vi "CleanHandler.ProcDestructor.vi"(0 "i ref in":refnum<vi>, 3 "ms timeout (100)":i32=100, 5 "error in (no error)":errorcluster) -> (14 "i ref out":refnum<vi>, 17 "timed out":bool, 19 "error out":errorcluster)   [LabVIEW 2014, in "CleanHandler.lvlib"]
doc: "This is the counterpart to ProcConstructor and is called befor the \"deactivate\" is called. This can be used to shutdown/deinitialize things."
uses:
  CleanHandler.lvlib
  CSCore/CSSystem/CoreDefs/CoreDefs.error_type.ctl
  CSCore/CSSystem/CoreLib/CoreLib.string 2 byte array.vi
  CSCore/CSSystem/CoreLib/CoreLib.lvlib
  CSCore/BaseProcess/BaseProcess.lvlib
  CSCore/CSSystem/CSSystemLib/CSSystemLib.lvlib
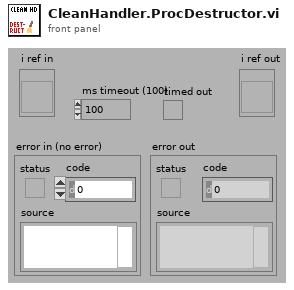
[diagram p1: front panel]
types:
  T1 = typedef "CoreDefs.error_type.ctl" = enum16{"no error", "can't load process", "can't unload process", "process does not exist", "can't install process", "can't remove process", "unknown function", "time out", "can't execute function", "duplicate queue name", "super not found", "caller queue invalid", "can't ping process", "unknown error", "VISA Error", "VISA timeout", "GPIB timeout", "GPIB error", "communication error", "data type mismatch", "can't read data from OPC server", "can't write data to OPC server", "OET error", "function not implemented", "process already exists", "invalid Shared Variable name", "error writing Shared Variable", "error reading Shared Variable", "invalid client name", "corrupt database", "unknown class", "call not authorized", "parameter out of range", "OET timeout: can't get data to modify", "invalid queue name", "requested operation incompatible with current state", "event undefined", "event disabled", "state undefined", "caller is not a friend", "EventBuilder: bad eventID", "EventBuilder: no DAQ devices", "a thread must not stop itself", "UNUSED ELEMENT4", "DiscArchiver: eventData incomplete", "DiscArchiver: eventData does not belong to run", "DiscArchiver: can't open file", "DiscArchiver: can't write to file", "DiscArchiver: available disc space low", "can't acquire semaphore", "error reading data from database", "notifier object is not existing", "can't register process", "can't unregister process", "illegal event type", "object disabled", "object already exists", "can't change state", "Instrument not found", "no connection to remote node", "invalid reference", "N/A", "UNUSED ELEMENT 1", "element not found", "illegal TCP/IP connection detected", "object does not exist", "invalid access ID", "unknown CS system", "invalid privilige", "unsupported data type", "unsupported server type", "IO server already exists", "Shared Variable already exists"}
  T2 = enum16{"simple", "synchronous", "asynchronous", "notification"}
  T3 = typedef "CoreDefs.rawDataType.ctl" = i8[]
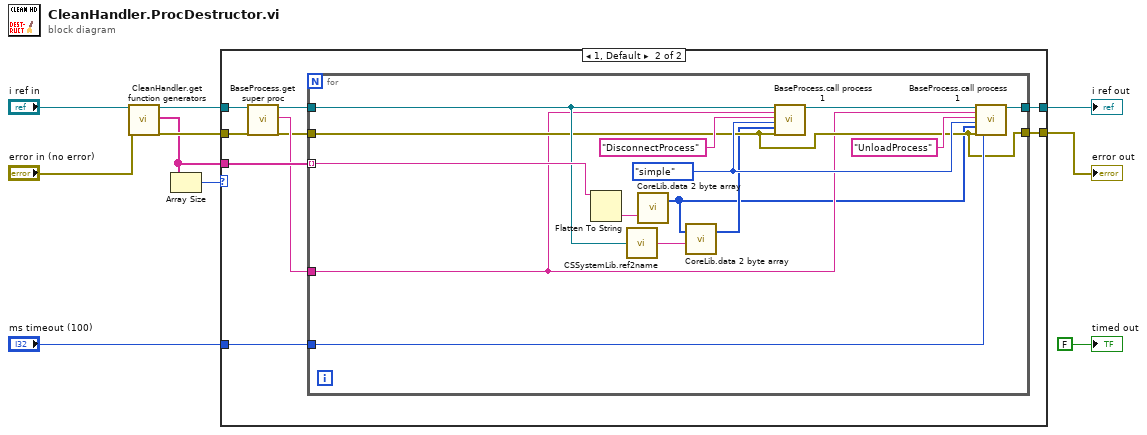
[diagram p0: block diagram]
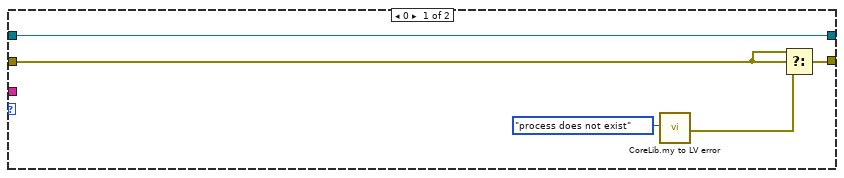
[diagram p2: hidden frame]
diagram:
  n1 = call "CleanHandler.get function generators.vi"("i ref in"="i ref in", "error in (no error)"="error in (no error)") -> ("i ref out"=w9:refnum<vi>, "function generators"=w7:string[], "error out"=w8:errorcluster)  [unwired: 14 in, 1 out]
  n2 = Array Size(array=w7) -> (size(s)=w10:i32)
  n3 = case shown="1, Default" w10 {
    tunnel: w9 -> [w15 w24]
    tunnel: w8 -> [w13 w23]
    tunnel: w7 -> [_ w21]
    tunnel: "ms timeout (100)" -> [_ w19]
    tunnel: [w14 w16] -> w1
    tunnel: [w15 w18] -> w2
    frame 0 {
      n4 = call "CoreLib.my to LV error.vi"("ErrorTypes"=CoreDefs.error_type."process does not exist") -> ("myErrorCluster"=w12:errorcluster)  [unwired: 17 in, 1 out]
      n5 = Select(t=w13, s=w13, f=w12) -> (s? t:f=w14:errorcluster)
    }
    frame 1, Default {
      n6 = call "BaseProcess.get super proc.vi"("i ref in"=w24, "error in (no error)"=w23) -> ("i ref out"=w22:refnum<vi>, "SuperProc"=w20:string, "error out"=w17:errorcluster)  [unwired: 15 in]
      n7 = for {
        tunnel: w22 -> [w31]
        tunnel: w21 -> [w37] mode=indexing
        tunnel: w20 -> [w29]
        tunnel: w19 -> [w33]
        tunnel: [w34] -> w18
        tunnel: w17 -> [w30]
        tunnel: [w30] -> w16
        w36 = T2."simple" ("CallType")
        n8 = Flatten To String(anything=w37) -> (data string=w28:string)  [unwired: 3 in, 2 out]
        n9 = call "CSSystemLib.ref2name.vi"("obj refnum"=w31) -> ("name"=w27:string)
        n10 = call-poly "CoreLib.data 2 byte array.vi"("string"=w28) -> ("byteArray out"=w25:T3)  [unwired: 18 in]
        n11 = call-poly "CoreLib.data 2 byte array.vi"("byteArray"=w25, "string"=w27) -> ("byteArray out"=w26:T3)  [unwired: 17 in]
        n12 = call "BaseProcess.call process 1.vi"("i ref in"=w31, "Object"=w29, "Selector"="DisconnectProcess", "CallType"=w36, "Data"=w26, "error in (no error)"=w30) -> ("i ref out"=w32:refnum<vi>)  [unwired: 11 in, 2 out]
        n13 = call "BaseProcess.call process 1.vi"("i ref in"=w32, "Object"=w29, "Selector"="UnloadProcess", "CallType"=w36, "Data"=w25, "error in (no error)"=w30, "timeout (ms)"=w33) -> ("i ref out"=w34:refnum<vi>)  [unwired: 10 in, 2 out]
      }
    }
  }
  "error out" <- w1
  "i ref out" <- w2
  "timed out" <- FALSE ("timed out")
